vi "Simple TCP - Server_20211123.vi"(8 "error in":errorcluster, 11 "TCP_Q":refnum<queue>) -> (0 "error out":errorcluster, 2 "TCP Connection":bool)   [LabVIEW 2018]
doc: "Demonstrates how to set up a basic TCP connection, send data to the specified port once a connection has been established, and terminate the connection once the data has been sent. This VI is designed to stop if the TCP connection is terminated. The data sent in this example is an array of random numbers."
uses:
  Controls/Enums/TCP_Loop.ctl
  Controls/Enums/WatchdogTimer_Enum.ctl
panel:
  out "TCP_Loop":i32
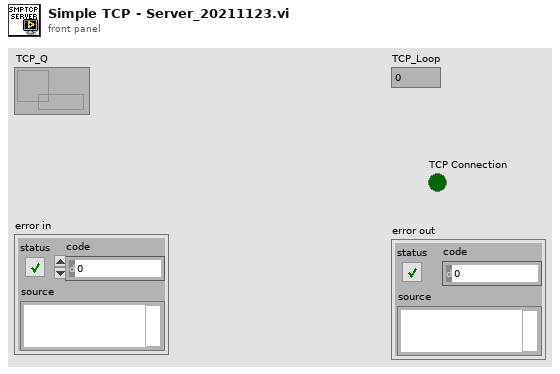
[diagram p1: front panel]
types:
  T1 = typedef "WatchdogTimer_Enum.ctl" = enum16{"ResetAll", "CheckAll", "HW1", "HW2", "Tones", "FP", "Noise", "Log", "TCP", "AI", "TC", "ADAM", "Disdrom", "TE", "Weather"}
  T2 = typedef "TCP_Loop.ctl" = enum16{"TCP_Write", "TCP_ChkTime", "TCP_Exit"}
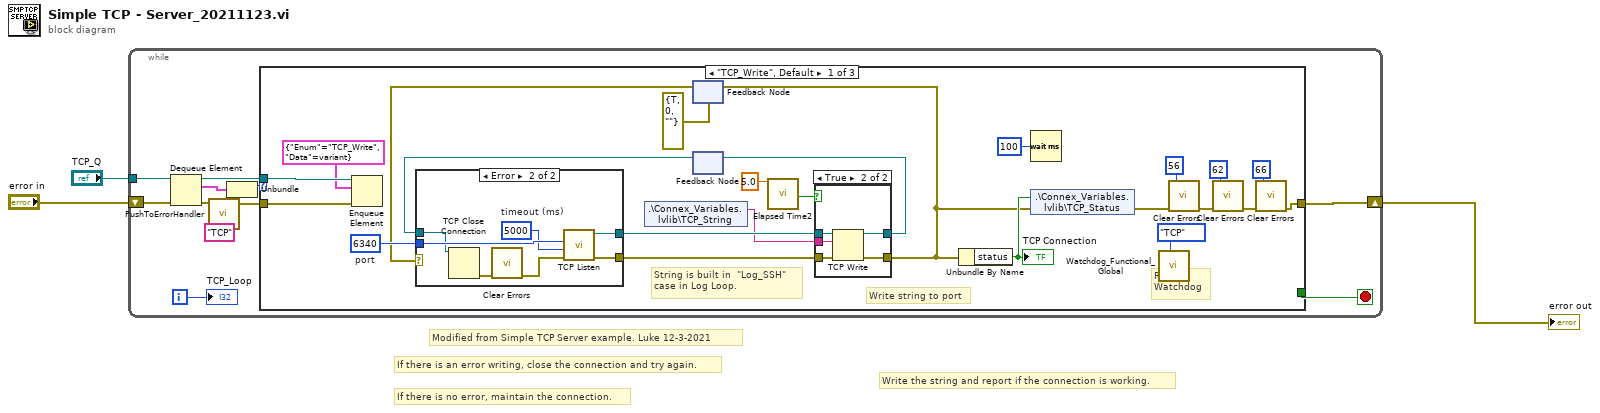
[diagram p0: block diagram]
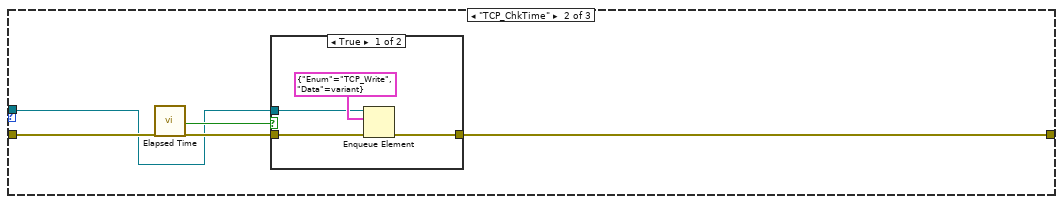
[diagram p4: hidden frame]
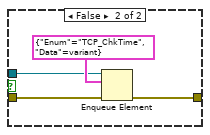
[diagram p5: hidden frame]
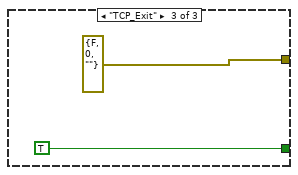
[diagram p6: hidden frame]
diagram:
  # "Modified from Simple TCP Server example. Luke 12-3-2021"
  # "Write the string and report if the connection is working."
  # "If there is no error, maintain the connection."
  # "If there is an error writing, close the connection and try again."
  n1 = while {
    tunnel: "TCP_Q" -> [w12]
    shift-right: [w6] -> w2
    shift-left: "error in" -> [w7]
    i -> [w13]
    stop <- w14 stop-if-true
    n2 = Dequeue Element(queue=w12, error in (no error)=w7) -> (queue out=w4:refnum<queue>, element=w11:cluster{"Enum":T2, "Data":variant}, error out=w9:errorcluster)  [unwired: 1 in, 1 out]
    n3 = call "PushToErrorHandler.vi"("ErrorIn"=w9, "ErrorLocation"="TCP") -> ("ErrorOut"=w5:errorcluster)  [unwired: 5 in]
    n4 = Unbundle(w11) -> ("Enum"=w10:T2)  [unwired: 1 out]
    n5 = case shown="\"TCP_Write\", Default" w10 {
      tunnel: [_ _ TRUE ("stop")] -> w14
      tunnel: [w18 w59 errorcluster {"status"=FALSE, "code"=0, "source"=""} ("error IO")] -> w6
      tunnel: w5 -> [w26 w56 _]
      tunnel: w4 -> [w25 w55 _]
      frame "TCP_Write", Default {
        w38 = u16 6340  # port
        # "String is built in  \"Log_SSH\" \ncase in Log Loop."
        # "Reset\nWatchdog"
        # "Write string to port"
        n6 = Enqueue Element(queue=w25, element=cluster{"Enum":T2, "Data":variant} {"Enum"=enum."TCP_Write", "Data"=variant}, error in (no error)=w26) -> ()  [unwired: 1 in, 3 out]
        n7 = shared-variable ".\\Connex_Variables.lvlib\\TCP_String"() -> (w31:string)  [unwired: 1 in, 1 out]
        n8 = feedback #1(errorcluster {"status"=TRUE, "code"=0, "source"=""} ("error out")) -> (w27:errorcluster)
        n9 = feedback #2() -> (w34:refnum<k5>)  [unwired: 1 in]
        n10 = case shown="Error" w27 {
          selector: w27 -> [w46 _]
          tunnel: w38 -> [_ w54]
          tunnel: [w46 w53] -> w37
          tunnel: [w47 w52] -> w36
          tunnel: w34 -> [w47 w51]
          frame No Error {
          }
          frame Error {
            w48 = 5000  # timeout (ms)
            n11 = TCP Close Connection(connection ID=w51) -> (error out=w50:errorcluster)  [unwired: 1 in, 2 out]
            n12 = call <vilib>:"Clear Errors.vi"("error in (no error)"=w50) -> ("error out"=w49:errorcluster)  [unwired: 5 in, 1 out]
            n13 = call <vilib>:"TCP Listen.vi"("error in (no error)"=w49, "timeout ms (wait forever: -1)"=w48, "port"=w54) -> ("error out"=w53:errorcluster, "connection ID"=w52:refnum<k5>)  [unwired: 4 in, 3 out]
          }
        }
        n14 = call "Elapsed Time2"("Time Target (s)"=5.0) -> ("Time has Elapsed"=w17:bool)  [unwired: 11 in, 7 out]
        n15 = case shown="True" w17 {
          tunnel: w37 -> [w39 w45]
          tunnel: w36 -> [w40 w44]
          tunnel: [w40 w43] -> w35
          tunnel: w31 -> [_ w42]
          tunnel: [w39 w41] -> w28
          frame False {
          }
          frame True {
            n16 = TCP Write(connection ID=w44, data in=w42, error in (no error)=w45) -> (connection ID out=w43:refnum<k5>, error out=w41:errorcluster)  [unwired: 2 out]
          }
        }
        n17 = feedback-in #1(w28) -> ()
        n18 = feedback-in #2(w35) -> ()
        n19 = Unbundle By Name(w28) -> ("status"=w30:bool)
        "TCP Connection" <- w30
        n20 = Wait (ms)(milliseconds to wait=u32 100) -> ()  [unwired: 1 out]
        n21 = shared-variable ".\\Connex_Variables.lvlib\\TCP_Status"(w30, error in=w28) -> (error out=w29:errorcluster)
        n22 = call "Watchdog_Functional_Global.vi"("Watchdog"=WatchdogTimer_Enum."TCP") -> ()  [unwired: 9 in, 2 out]
        n23 = call <vilib>:"Clear Errors.vi"("error in (no error)"=w29, "specific error code to clear (0: all)"=56) -> ("error out"=w21:errorcluster)  [unwired: 4 in, 1 out]
        n24 = call <vilib>:"Clear Errors.vi"("error in (no error)"=w21, "specific error code to clear (0: all)"=62) -> ("error out"=w19:errorcluster)  [unwired: 4 in, 1 out]
        n25 = call <vilib>:"Clear Errors.vi"("error in (no error)"=w19, "specific error code to clear (0: all)"=66) -> ("error out"=w18:errorcluster)  [unwired: 4 in, 1 out]
      }
      frame "TCP_ChkTime" {
        n26 = call "Elapsed Time"("error in (no error)"=w56) -> ("Time has Elapsed"=w58:bool, "error out"=w57:errorcluster)  [unwired: 11 in, 6 out]
        n27 = case shown="True" w58 {
          tunnel: w55 -> [w62 w66]
          tunnel: w57 -> [w61 w65]
          tunnel: [w60 w64] -> w59
          frame True {
            n28 = Enqueue Element(queue=w62, element=cluster{"Enum":T2, "Data":variant} {"Enum"=enum."TCP_Write", "Data"=variant}, error in (no error)=w61) -> (error out=w60:errorcluster)  [unwired: 1 in, 2 out]
          }
          frame False {
            n29 = Enqueue Element(queue=w66, element=cluster{"Enum":T2, "Data":variant} {"Enum"=enum."TCP_ChkTime", "Data"=variant}, error in (no error)=w65) -> (error out=w64:errorcluster)  [unwired: 1 in, 2 out]
          }
        }
      }
      frame "TCP_Exit" {
      }
    }
    "TCP_Loop" <- w13
  }
  "error out" <- w2
